vi "MIDDLE.vi"(8 "PUMPS ON/OFF":bool, 9 "HAND/AUTO":bool, 10 "SYSTEM ON/OFF":bool, 11 "EMERGENCY ON/OFF":bool) -> (0 "Tasks":string, 3 "State":string)   [LabVIEW 2014]
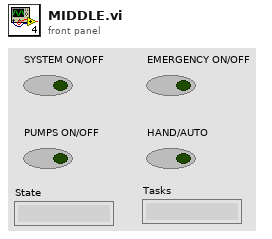
[diagram p1: front panel]
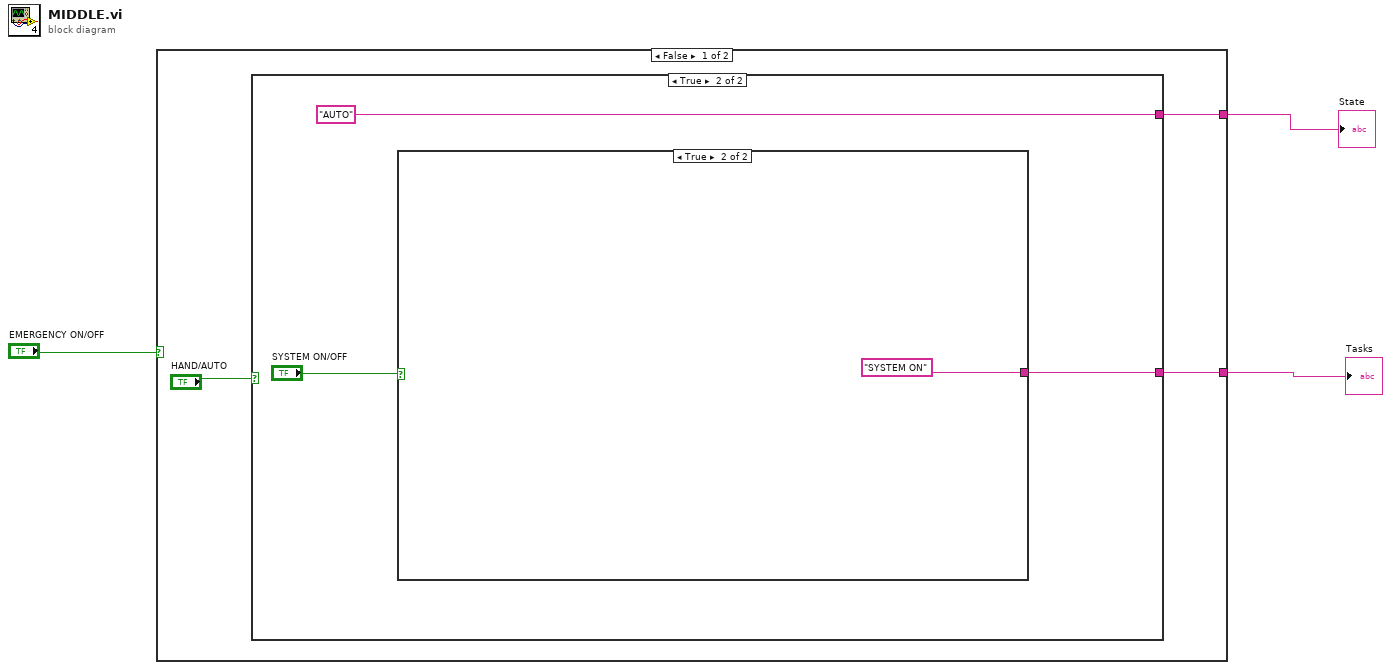
[diagram p0: block diagram]
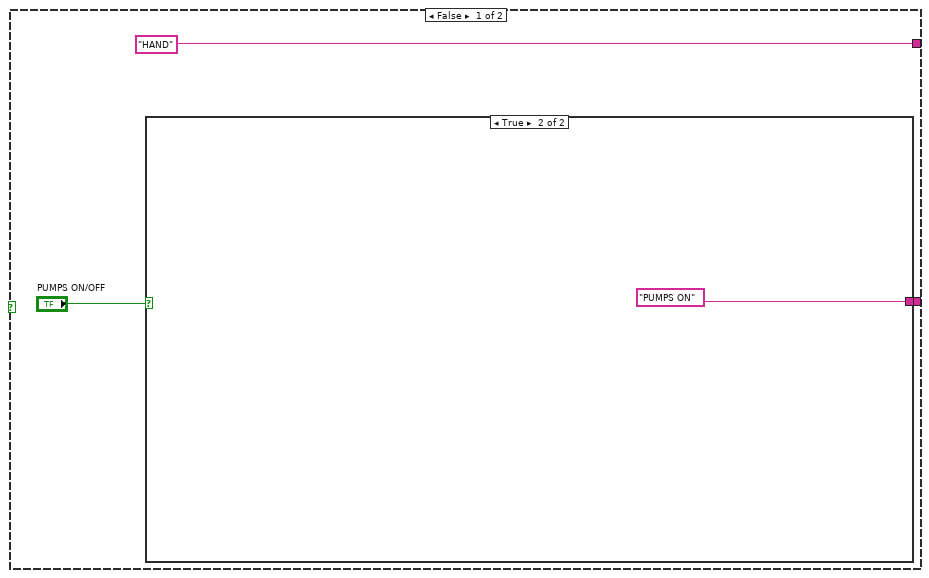
[diagram p2: hidden frame]
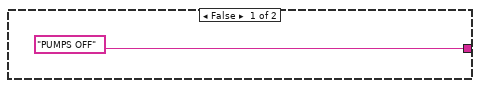
[diagram p3: hidden frame]
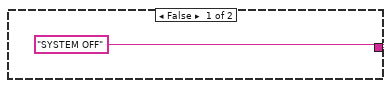
[diagram p4: hidden frame]
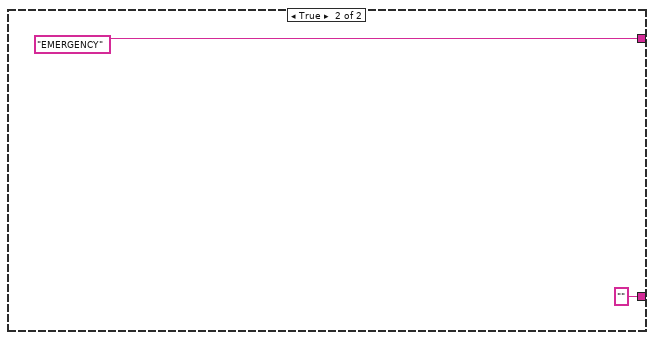
[diagram p5: hidden frame]
diagram:
  n1 = case shown="False" "EMERGENCY ON/OFF" {
    tunnel: [w5 "EMERGENCY"] -> w2
    tunnel: [w4 ""] -> w1
    frame False {
      n2 = case shown="True" "HAND/AUTO" {
        tunnel: ["HAND" "AUTO"] -> w5
        tunnel: [w7 w12] -> w4
        frame False {
          n3 = case shown="True" "PUMPS ON/OFF" {
            tunnel: ["PUMPS OFF" "PUMPS ON"] -> w7
            frame False {
            }
            frame True {
            }
          }
        }
        frame True {
          n4 = case shown="True" "SYSTEM ON/OFF" {
            tunnel: ["SYSTEM OFF" "SYSTEM ON"] -> w12
            frame False {
            }
            frame True {
            }
          }
        }
      }
    }
    frame True {
    }
  }
  "State" <- w2
  "Tasks" <- w1
